vi "4 wire measurements_make before break.vi"(4 "5":string(combo)="NC", 5 "26":string(combo)="NC", 6 "4":string(combo)="NC", 7 "27":string(combo)="y1", 8 "3":string(combo)="NC", 9 "2":string(combo)="y5", 10 "1":string(combo)="y3", 11 "28":string(combo)="y4") -> ()   [LabVIEW 2011]
panel:
  in  "Disconnect all?":bool
  in  "IVI Option String":string="Simulate=0,RangeCheck=1,QueryInstrStatus=0,Cache=1,DriverSetup=Model:40-726-511;"
  in  "VISA Resource Name":string="PXI9::13::INSTR"
  in  "X Channel Ground":string="x12"
  in  "Discharge Y Channels?":bool=TRUE
  in  "Discharge X channels?":bool=TRUE
  in  "Y Channel Ground":string="y1"
  # "4 wire              measurements\n\nNotes:\nLock-in 1: I+/I- -->AO0/AI0, board 0\n\nLock-in 3: V+/V-  --> AI0, board 1.  \n  V+/V- conencted to y3 and y4. OSC output should set the same as Lock-in 1\n\nLock-in 2: I2+/I2- -->AO1/AI1, board 0"
  # "1"
  # "28"
  # "27"
  # "26"
  # "2"
  # "3"
  # "4"
  # "The numbers correspond to the \nchip socket. \nMake sure schematic is accurate."
  # "!"
  # "5"
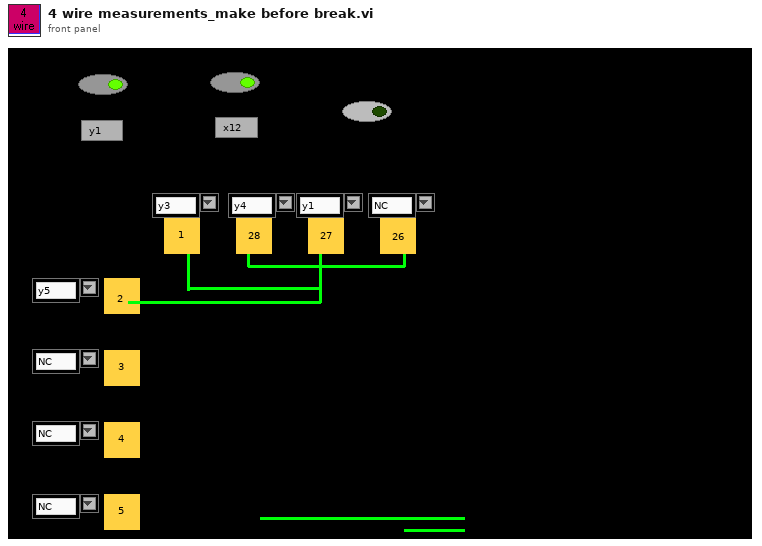
[diagram p1: front panel]
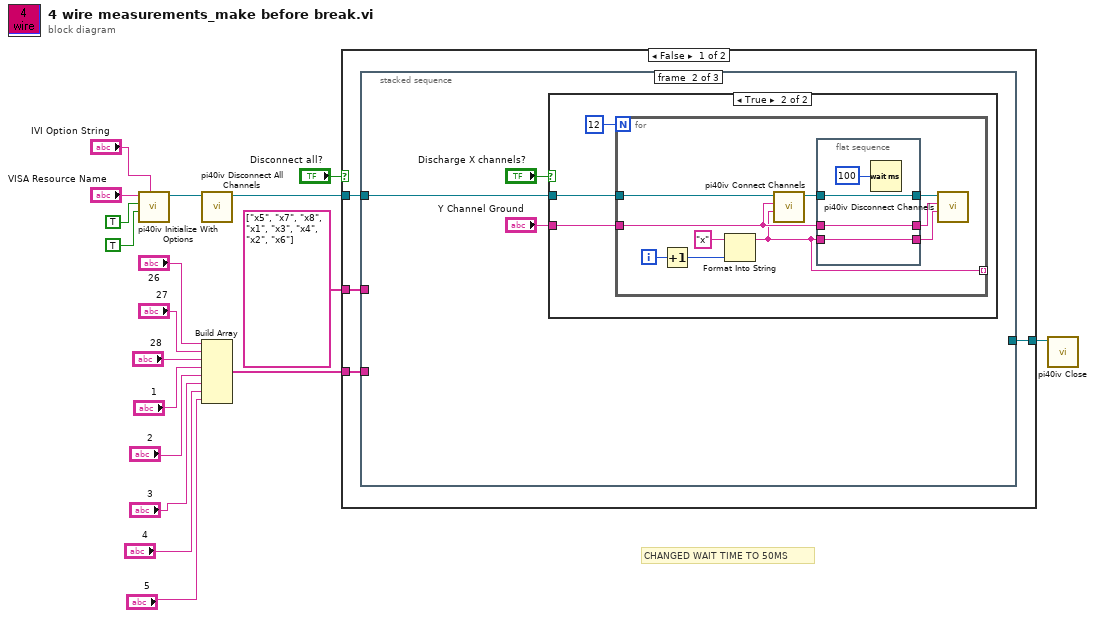
[diagram p0: block diagram]
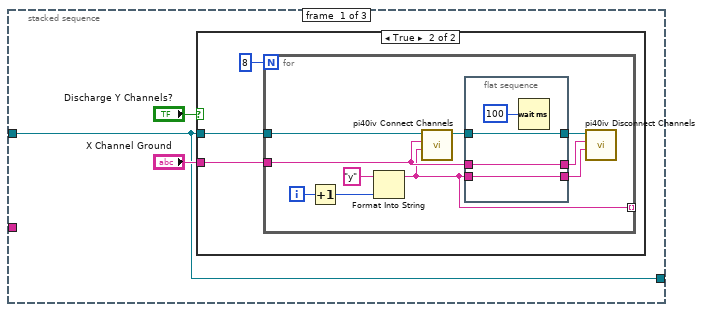
[diagram p2: hidden frame]
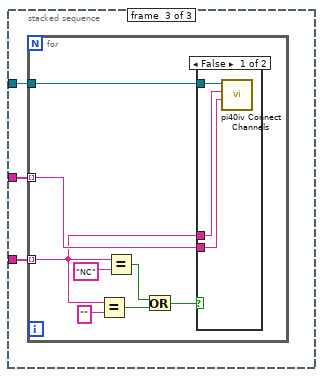
[diagram p5: hidden frame]
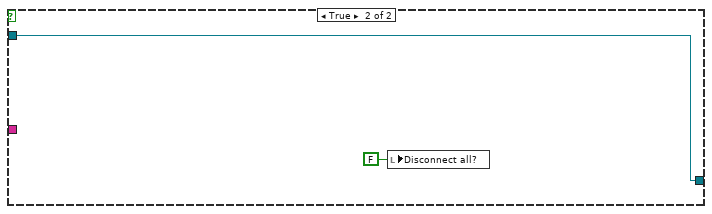
[diagram p7: hidden frame]
diagram:
  # "CHANGED WAIT TIME TO 50MS"
  n1 = call <instrlib>:"pi40iv Initialize With Options.vi"("option string"="IVI Option String", "reset device"=TRUE, "id query"=TRUE, "resource name"="VISA Resource Name") -> ("instrument handle out"=w10:refnum<k15>)  [unwired: 6 in, 1 out]
  n2 = call <instrlib>:"pi40iv Disconnect All Channels.vi"("instrument handle"=w10) -> ("instrument handle out"=w9:refnum<k15>)  [unwired: 9 in, 1 out]
  n3 = Build Array("26", "27", "28", "1", "2", "3", "4", "5") -> (w12:string[])
  n4 = case shown="False" "Disconnect all?" {
    tunnel: w12 -> [w22 _]
    tunnel: string[] ["x5", "x7", "x8", "x1", "x3", "x4", "x2", "x6"] -> [w21 _]
    tunnel: w9 -> [w20 w78]
    tunnel: [w19 w78] -> w7
    frame False {
      n5 = stacked-sequence {
        tunnel: w20 -> [w23 w45 w65]
        tunnel: w22 -> [_ _ w64]
        tunnel: w21 -> [_ _ w63]
        tunnel: [w23 _ _] -> w19
        frame #0 {
          n6 = case shown="True" "Discharge Y Channels?" {
            tunnel: w23 -> [_ w28]
            tunnel: "X Channel Ground" -> [_ w27]
            frame False {
            }
            frame True {
              n7 = for {
                N: 8 -> [_]
                tunnel: w28 -> [w38]
                tunnel: w27 -> [w35]
                tunnel: [w30] -> _ mode=indexing
                i -> [w31]
                n8 = Increment(x=w31) -> (x+1=w29:i32)
                n9 = Format Into String(initial string="y", w29) -> (resulting string=w30:string)  [unwired: 2 in, 1 out]
                n10 = call <instrlib>:"pi40iv Connect Channels.vi"("channel 2"=w30, "channel 1"=w35, "instrument handle"=w38) -> ("instrument handle out"=w37:refnum<k15>)  [unwired: 7 in, 1 out]
                n11 = flat-sequence {
                  tunnel: w37 -> [w42]
                  tunnel: [w42] -> w36
                  tunnel: w35 -> [w40]
                  tunnel: [w40] -> w34
                  tunnel: w30 -> [w39]
                  tunnel: [w39] -> w33
                  frame #0 {
                    n12 = Wait (ms)(milliseconds to wait=u32 100) -> ()  [unwired: 1 out]
                  }
                }
                n13 = call <instrlib>:"pi40iv Disconnect Channels.vi"("channel 2"=w33, "channel 1"=w34, "instrument handle"=w36) -> ()  [unwired: 7 in, 2 out]
              }
            }
          }
        }
        frame #1 {
          n14 = case shown="True" "Discharge X channels?" {
            tunnel: w45 -> [_ w48]
            tunnel: "Y Channel Ground" -> [_ w47]
            frame False {
            }
            frame True {
              n15 = for {
                N: 12 -> [_]
                tunnel: w48 -> [w58]
                tunnel: w47 -> [w55]
                tunnel: [w50] -> _ mode=indexing
                i -> [w51]
                n16 = Increment(x=w51) -> (x+1=w49:i32)
                n17 = Format Into String(initial string="x", w49) -> (resulting string=w50:string)  [unwired: 2 in, 1 out]
                n18 = call <instrlib>:"pi40iv Connect Channels.vi"("channel 2"=w50, "channel 1"=w55, "instrument handle"=w58) -> ("instrument handle out"=w57:refnum<k15>)  [unwired: 7 in, 1 out]
                n19 = flat-sequence {
                  tunnel: w57 -> [w62]
                  tunnel: [w62] -> w56
                  tunnel: w55 -> [w60]
                  tunnel: [w60] -> w54
                  tunnel: w50 -> [w59]
                  tunnel: [w59] -> w53
                  frame #0 {
                    n20 = Wait (ms)(milliseconds to wait=u32 100) -> ()  [unwired: 1 out]
                  }
                }
                n21 = call <instrlib>:"pi40iv Disconnect Channels.vi"("channel 2"=w53, "channel 1"=w54, "instrument handle"=w56) -> ()  [unwired: 7 in, 2 out]
              }
            }
          }
        }
        frame #2 {
          n22 = for {
            tunnel: w65 -> [w73]
            tunnel: w64 -> [w66] mode=indexing
            tunnel: w63 -> [w67] mode=indexing
            n23 = Equal?(x=w66, y="") -> (x = y?=w69:bool)
            n24 = Equal?(x=w66, y="NC") -> (x = y?=w71:bool)
            n25 = Or(x=w71, y=w69) -> (x .or. y?=w70:bool)
            n26 = case shown="False" w70 {
              tunnel: w73 -> [w76 _]
              tunnel: w67 -> [w75 _]
              tunnel: w66 -> [w74 _]
              frame False {
                n27 = call <instrlib>:"pi40iv Connect Channels.vi"("channel 2"=w75, "channel 1"=w74, "instrument handle"=w76) -> ()  [unwired: 7 in, 2 out]
              }
              frame True {
              }
            }
          }
        }
      }
    }
    frame True {
      n28 = local write "Disconnect all?"(FALSE ("Disconnect all?")) -> ()
    }
  }
  n29 = call <instrlib>:"pi40iv Close.vi"("instrument handle"=w7) -> ()  [unwired: 10 in, 1 out]
